vi "operation.vi"(6 "operation":T1=enum."T+", 7 "clear buffer (F)":bool, 8 "error in (no error)":errorcluster, 10 "cube":refnum<vi>, 11 "cube in":T2) -> (0 "error out":errorcluster, 3 "cube out":T2)   [LabVIEW 2011]
uses:
  Typedef/cube.ctl
  Typedef/face.ctl
  Typedef/operation.ctl
  Typedef/cube rotate direction.ctl
panel:
  out "number of operations":i32
  out "operations":T1[](array[typedef])
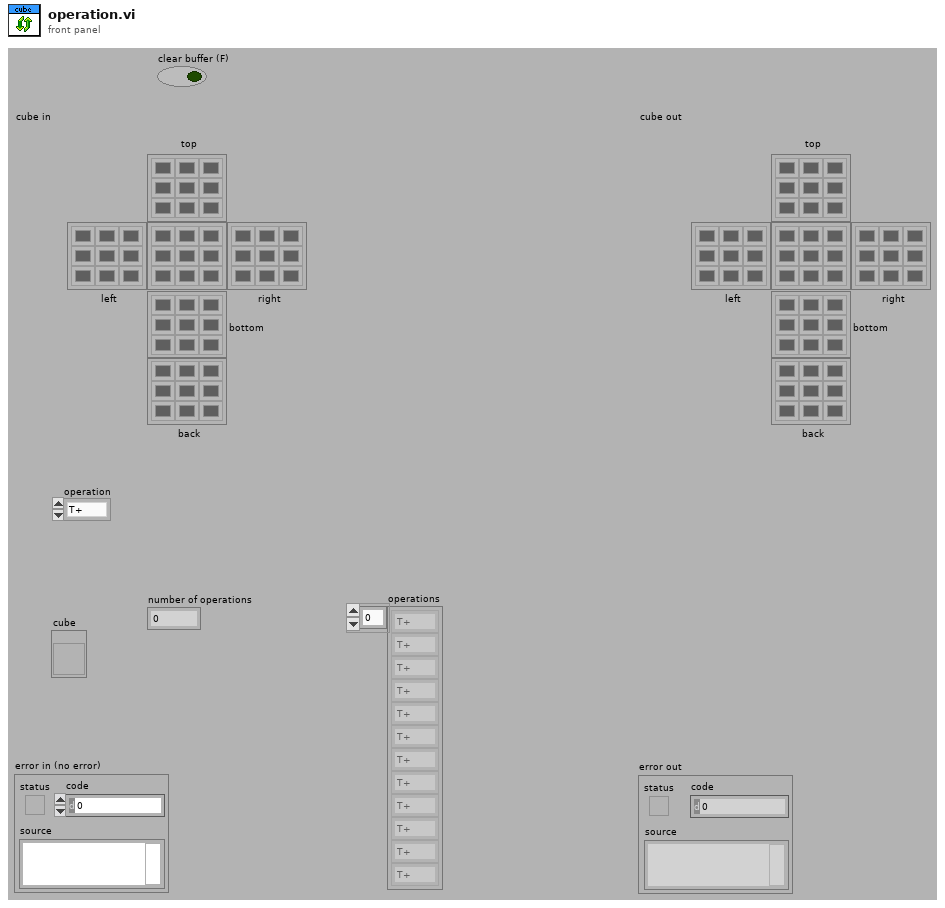
[diagram p1: front panel]
types:
  T1 = typedef "operation.ctl" = enum16{"nop", "T+", "T-", "F+", "F-", "L+", "L-", "R+", "R-", "B+", "B-", "<--", "-->", "^", "V"}
  T2 = typedef "cube.ctl" = cluster{"top":T3, "left":T3, "right":T3, "bottom":T3, "back":T3, "front":T3}
  T3 = typedef "face.ctl" = u32[][]
  T4 = typedef "cube rotate direction.ctl" = enum16{"up", "down", "left", "right"}
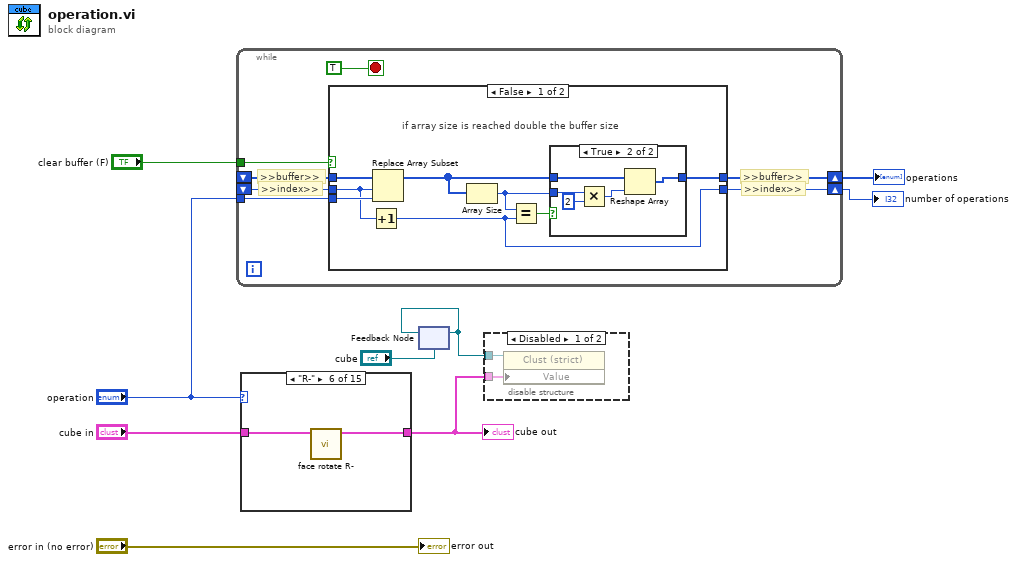
[diagram p0: block diagram]
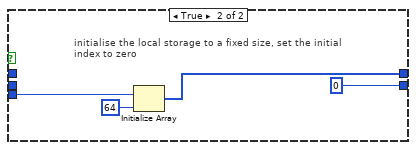
[diagram p4: hidden frame]
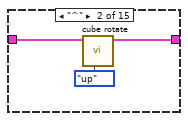
[diagram p6: hidden frame]
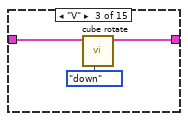
[diagram p7: hidden frame]
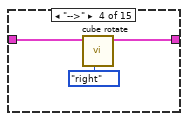
[diagram p8: hidden frame]
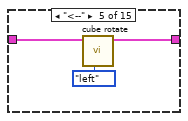
[diagram p9: hidden frame]
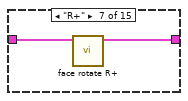
[diagram p10: hidden frame]
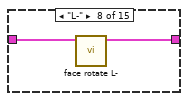
[diagram p11: hidden frame]
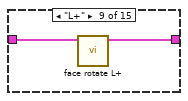
[diagram p12: hidden frame]
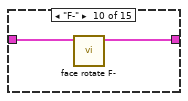
[diagram p13: hidden frame]
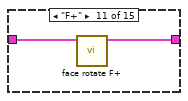
[diagram p14: hidden frame]
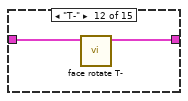
[diagram p15: hidden frame]
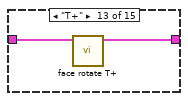
[diagram p16: hidden frame]
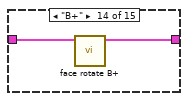
[diagram p17: hidden frame]
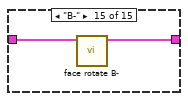
[diagram p18: hidden frame]
diagram:
  n1 = while {
    tunnel: "operation" -> [w16]
    shift-right: [w15] -> w5
    shift-left: _ -> [w14]
    tunnel: "clear buffer (F)" -> [w13]
    shift-right: [w11] -> w4
    shift-left: _ -> [w10]
    stop <- TRUE stop-if-true
    # ">>buffer>>"
    # ">>index>>"
    # ">>buffer>>"
    # ">>index>>"
    n2 = case shown="False" w13 {
      tunnel: w16 -> [w23 w34]
      tunnel: [w19 w33] -> w15
      tunnel: w14 -> [w24 _]
      tunnel: [w17 0 ("dimension size")] -> w11
      tunnel: w10 -> [w22 _]
      frame False {
        # "if array size is reached double the buffer size"
        n3 = Increment(x=w22) -> (x+1=w17:i32)
        n4 = Replace Array Subset(array=w24, new element=w23, index=w22) -> (w21:T1[])
        n5 = Array Size(array=w21) -> (size(s)=w20:i32)
        n6 = Equal?(x=w20, y=w17) -> (x = y?=w18:bool)
        n7 = case shown="True" w18 {
          tunnel: w21 -> [w25 w30]
          tunnel: w20 -> [_ w28]
          tunnel: [w25 w26] -> w19
          frame False {
          }
          frame True {
            n8 = Multiply(x=w28, y=2) -> (x*y=w29:i32)
            n9 = Reshape Array(w30, w29) -> (w26:T1[])
          }
        }
      }
      frame True {
        # "initialise the local storage to a fixed size, set the initial\nindex to zero"
        n10 = Initialize Array(w34, 64 ("dimension size")) -> (w33:T1[])
      }
    }
  }
  "operations" <- w5
  "number of operations" <- w4
  n11 = case shown="\"R-\"" "operation" {
    tunnel: [w35 w36 w39 w42 w45 w48 w50 w52 w54 w56 w58 w60 w62 w64 w66] -> w3
    tunnel: "cube in" -> [w35 w37 w40 w43 w46 w49 w51 w53 w55 w57 w59 w61 w63 w65 w67]
    frame "nop" {
    }
    frame "^" {
      n12 = call "cube rotate.vi"("cube rotation direction"=cube_rotate_direction."up", "cube in"=w37) -> ("cube out"=w36:T2)  [unwired: 8 in, 1 out]
    }
    frame "V" {
      n13 = call "cube rotate.vi"("cube rotation direction"=cube_rotate_direction."down", "cube in"=w40) -> ("cube out"=w39:T2)  [unwired: 8 in, 1 out]
    }
    frame "-->" {
      n14 = call "cube rotate.vi"("cube rotation direction"=cube_rotate_direction."right", "cube in"=w43) -> ("cube out"=w42:T2)  [unwired: 8 in, 1 out]
    }
    frame "<--" {
      n15 = call "cube rotate.vi"("cube rotation direction"=cube_rotate_direction."left", "cube in"=w46) -> ("cube out"=w45:T2)  [unwired: 8 in, 1 out]
    }
    frame "R-" {
      n16 = call "face rotate R-.vi"("cube in"=w49) -> ("cube out"=w48:T2)  [unwired: 9 in, 1 out]
    }
    frame "R+" {
      n17 = call "face rotate R+.vi"("cube in"=w51) -> ("cube out"=w50:T2)  [unwired: 9 in, 1 out]
    }
    frame "L-" {
      n18 = call "face rotate L-.vi"("cube in"=w53) -> ("cube out"=w52:T2)  [unwired: 9 in, 1 out]
    }
    frame "L+" {
      n19 = call "face rotate L+.vi"("cube in"=w55) -> ("cube out"=w54:T2)  [unwired: 9 in, 1 out]
    }
    frame "F-" {
      n20 = call "face rotate F-.vi"("cube in"=w57) -> ("cube out"=w56:T2)  [unwired: 9 in, 1 out]
    }
    frame "F+" {
      n21 = call "face rotate F+.vi"("cube in"=w59) -> ("cube out"=w58:T2)  [unwired: 9 in, 1 out]
    }
    frame "T-" {
      n22 = call "face rotate T-.vi"("cube in"=w61) -> ("cube out"=w60:T2)  [unwired: 9 in, 1 out]
    }
    frame "T+" {
      n23 = call "face rotate T+.vi"("cube in"=w63) -> ("cube out"=w62:T2)  [unwired: 9 in, 1 out]
    }
    frame "B+" {
      n24 = call "face rotate B+.vi"("cube in"=w65) -> ("cube out"=w64:T2)  [unwired: 9 in, 1 out]
    }
    frame "B-" {
      n25 = call "face rotate B-.vi"("cube in"=w67) -> ("cube out"=w66:T2)  [unwired: 9 in, 1 out]
    }
  }
  "cube out" <- w3
  n26 = feedback #1("cube") -> (w1:refnum<vi>)
  n27 = feedback-in #1(w1) -> ()
  n28 = disable-structure shown="Disabled" {
    disable-tunnel: w3 -> [w69 _]
    disable-tunnel: w1 -> [w68 _]
    frame Disabled {
      n29 = property class="Clust (strict)"(reference=w68, "Value"=w69) -> ()  [unwired: 1 in, 2 out]
    }
    frame Enabled {
    }
  }
  "error out" <- "error in (no error)"
